vi "Disarm.vi"(8 "error in (no error)":errorcluster, 9 "Request type":T1=enum."User command", 11 "DAQmx Lockin Digitizer Driver in":refnum<class "DAQmx Lockin Digitizer Driver.lvclass">) -> (0 "error out":errorcluster, 2 "Armed":bool, 3 "DAQmx Lockin Digitizer Driver out":refnum<class "DAQmx Lockin Digitizer Driver.lvclass">)   [LabVIEW 2021, in "DAQmx Lockin Digitizer Driver.lvclass"]
uses:
  DAQmx Lockin Digitizer Driver.lvclass
  C:/GitHub/NHMFL_Core/Libraries/Instruments/Pulse Driver/Lockin Digitizer Driver/Lockin Digitizer Driver.lvclass
  C:/GitHub/NHMFL_Core/Libraries/Instruments/Pulse Driver/Pulse Driver.lvclass
  LabActor/Controllers/Process Controller/Request type.ctl
  DAQmx Lockin Driver/DAQmx Lockin Driver.lvclass
  DAQmx Lockin Digitizer Driver.lvclass/DAQmx Lockin Digitizer Driver.ctl
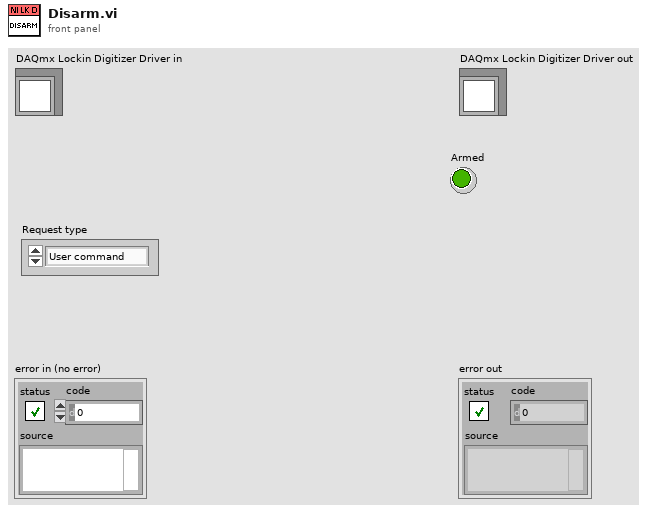
[diagram p1: front panel]
types:
  T1 = typedef "Request type.ctl" = enum16{"Process complete", "User command", "Auto-restart", "Error"}
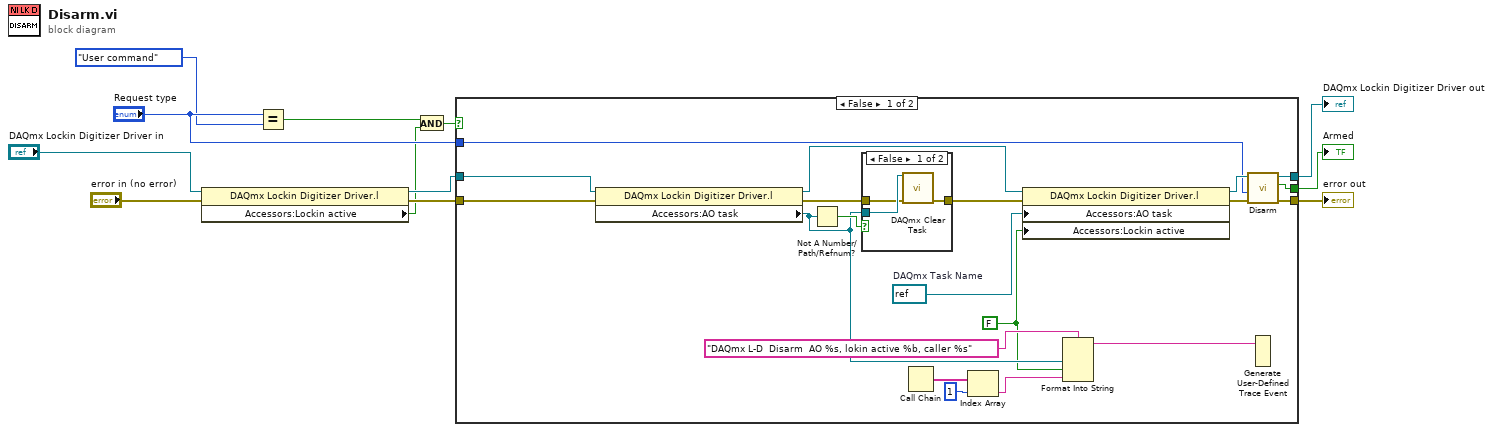
[diagram p0: block diagram]
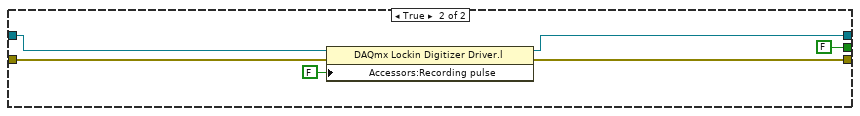
[diagram p3: hidden frame]
diagram:
  n1 = property class="DAQmx Lockin Digitizer Driver.l"(reference="DAQmx Lockin Digitizer Driver in", error in="error in (no error)") -> (reference out=w8:refnum<class "DAQmx Lockin Digitizer Driver.lvclass">, error out=w6:errorcluster, "Accessors:Lockin active"=w2:bool)
  n2 = Equal?(x="Request type", y=Request_type."User command") -> (x = y?=w3:bool)
  n3 = And(x=w3, y=w2) -> (x .and. y?=w1:bool)
  n4 = case shown="False" w1 {
    tunnel: [w32 w40] -> w12
    tunnel: [w31 FALSE ("Armed")] -> w11
    tunnel: [w30 w38] -> w10
    tunnel: w8 -> [w24 w39]
    tunnel: w6 -> [w23 w42]
    tunnel: "Request type" -> [w14 _]
    frame False {
      w13 = FALSE ("Lockin active")
      w18 = refnum<k21> refnum  # DAQmx Task Name
      n5 = property class="DAQmx Lockin Digitizer Driver.l"(reference=w24, error in=w23) -> (reference out=w29:refnum<class "DAQmx Lockin Digitizer Driver.lvclass">, error out=w27:errorcluster, "Accessors:AO task"=w19:refnum<k21>)
      n6 = Not A Number/Path/Refnum?(number/path/refnum=w19) -> (NaN/Path/Refnum?=w26:bool)
      n7 = case shown="False" w26 {
        tunnel: w19 -> [w35 _]
        tunnel: w27 -> [w34 w36]
        tunnel: [w33 w36] -> w28
        frame False {
          n8 = call <vilib>:"DAQmx Clear Task.vi"("task in"=w35, "error in"=w34) -> ("error out"=w33:errorcluster)  [unwired: 13 out]
        }
        frame True {
        }
      }
      n9 = Call Chain() -> (call chain=w17:string[])
      n10 = Index Array(array=w17, index=1) -> (element=w15:string)
      n11 = property class="DAQmx Lockin Digitizer Driver.l"(reference=w29, error in=w28, "Accessors:AO task"=w18, "Accessors:Lockin active"=w13) -> (reference out=w25:refnum<class "DAQmx Lockin Digitizer Driver.lvclass">, error out=w22:errorcluster)
      n12 = Format Into String(format string="DAQmx L-D  Disarm  AO %s, lokin active %b, caller %s" ("string"), w19, w13, w15) -> (resulting string=w20:string)  [unwired: 2 in, 1 out]
      n13 = call-parent "Disarm.vi"("error in (no error)"=w22, "Request type"=w14, "DAQmx Digitizer in"=w25) -> ("error out"=w32:errorcluster, "Armed"=w31:bool, "DAQmx Digitizer out"=w30:refnum<class "DAQmx Lockin Digitizer Driver.lvclass">)  [unwired: 6 in]
      n14 = Generate User-Defined Trace Event(2:w20) -> ()  [unwired: 1 in]
    }
    frame True {
      n15 = property class="DAQmx Lockin Digitizer Driver.l"(reference=w39, error in=w42, "Accessors:Recording pulse"=FALSE ("Recording pulse")) -> (reference out=w38:refnum<class "DAQmx Lockin Digitizer Driver.lvclass">, error out=w40:errorcluster)
    }
  }
  "error out" <- w12
  "DAQmx Lockin Digitizer Driver out" <- w10
  "Armed" <- w11
